vi "Write Roughness.vi"(8 "error in (no error)":errorcluster, 10 "Roughness":T1, 11 "Depth Data Message in":refnum<class "Depth Data Message.lvclass">) -> (0 "error out":errorcluster, 3 "Depth Data Message out":refnum<class "Depth Data Message.lvclass">)   [LabVIEW 2018, in "Depth Data Message.lvclass"]
uses:
  Depth Data Message.lvclass
  Depth Data Message.lvclass/Depth Data Message.ctl
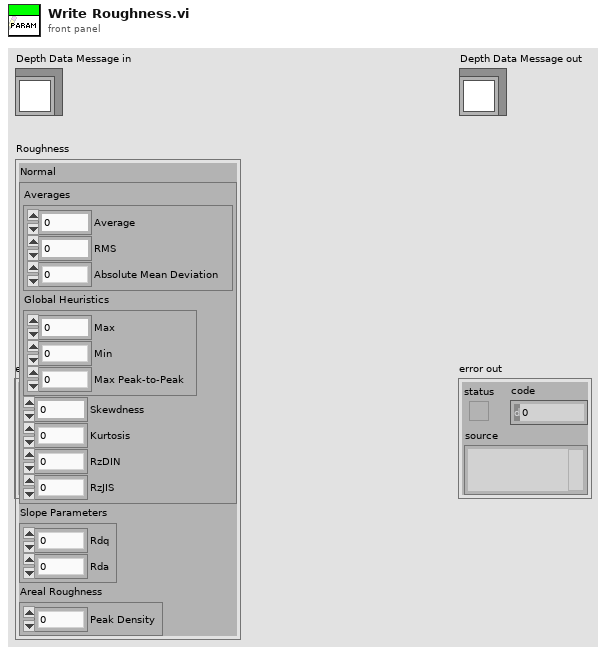
[diagram p1: front panel]
types:
  T1 = cluster{"Normal":cluster{"Averages":cluster{"Average":dbl, "RMS":dbl, "Absolute Mean Deviation":dbl}, "Global Heuristics":cluster{"Max":dbl, "Min":dbl, "Max Peak-to-Peak":dbl}, "Skewdness":dbl, "Kurtosis":dbl, "RzDIN":dbl, "RzJIS":dbl}, "Slope Parameters":cluster{"Rdq":dbl, "Rda":dbl}, "Areal Roughness":cluster{"Peak Density":dbl}}
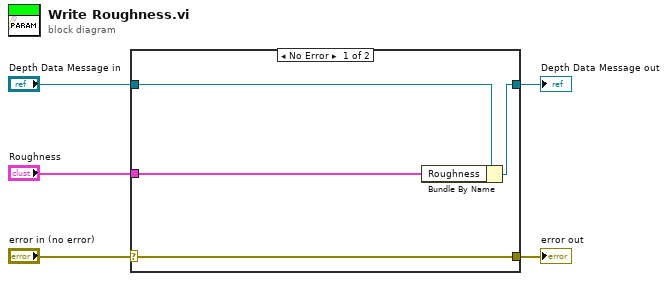
[diagram p0: block diagram]
diagram:
  n1 = case shown="No Error" "error in (no error)" {
    selector: "error in (no error)" -> [w9 w10]
    tunnel: [w9 w10] -> w4
    tunnel: [w7 w11] -> w2
    tunnel: "Depth Data Message in" -> [w8 w11]
    tunnel: "Roughness" -> [w6 _]
    frame No Error {
      n2 = Bundle By Name(cluster=w8, "Roughness"=w6) -> (w7:refnum<class "Depth Data Message.lvclass">)
    }
    frame Error {
    }
  }
  "error out" <- w4
  "Depth Data Message out" <- w2
